vi "Document My VI QuickDrop Plugin.vi"(6 "Variant in":variant, 7 "Shift Pressed?":bool, 8 "error in (no error)":errorcluster, 10 "QD Combo Box Ref":refnum<vi>, 11 "QD Launch VI Ref":refnum<vi>) -> (0 "error out":errorcluster, 4 "Variant out":variant)   [LabVIEW 2014]
doc: "This VI allows the VI Description Tool to be used with the Quick Drop Frame work\n\nDefault Shortcut - [A]"
uses:
  <userlib>/GA/VI Documentation Tool/TYPE_Version Status.ctl
panel:
  in  "Undo Name":string="Quick Drop Keyboard Shortcut"
  # "Do not change the connector pane of this VI.\n\nSee the block diagram for directions on how to use this template."
  # "Specify the name of the Undo transaction"
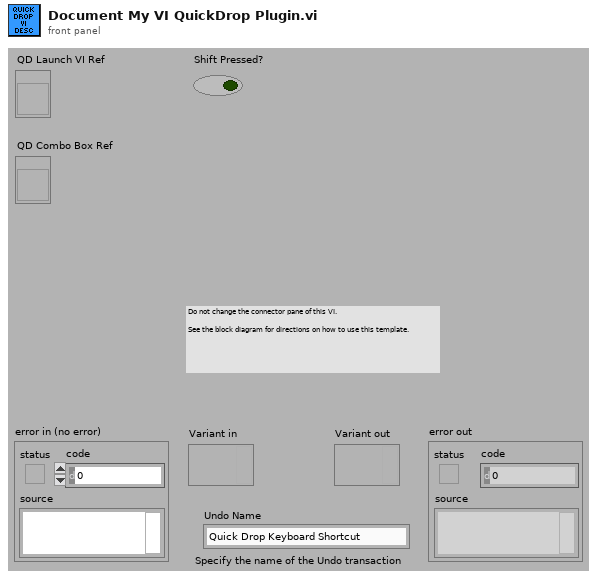
[diagram p1: front panel]
types:
  T1 = typedef "TYPE_Version Status.ctl" = enum16{"Development", "alpha", "beta", "Reviewed", "Bug", "Other"}
  T2 = typedef "TYPE_Description Cluster.ctl" = cluster{"VI Description":string, "VI Version":string, "Review Date":string, "Author":string, "Copyright":string, "Requirements Coverage":string}
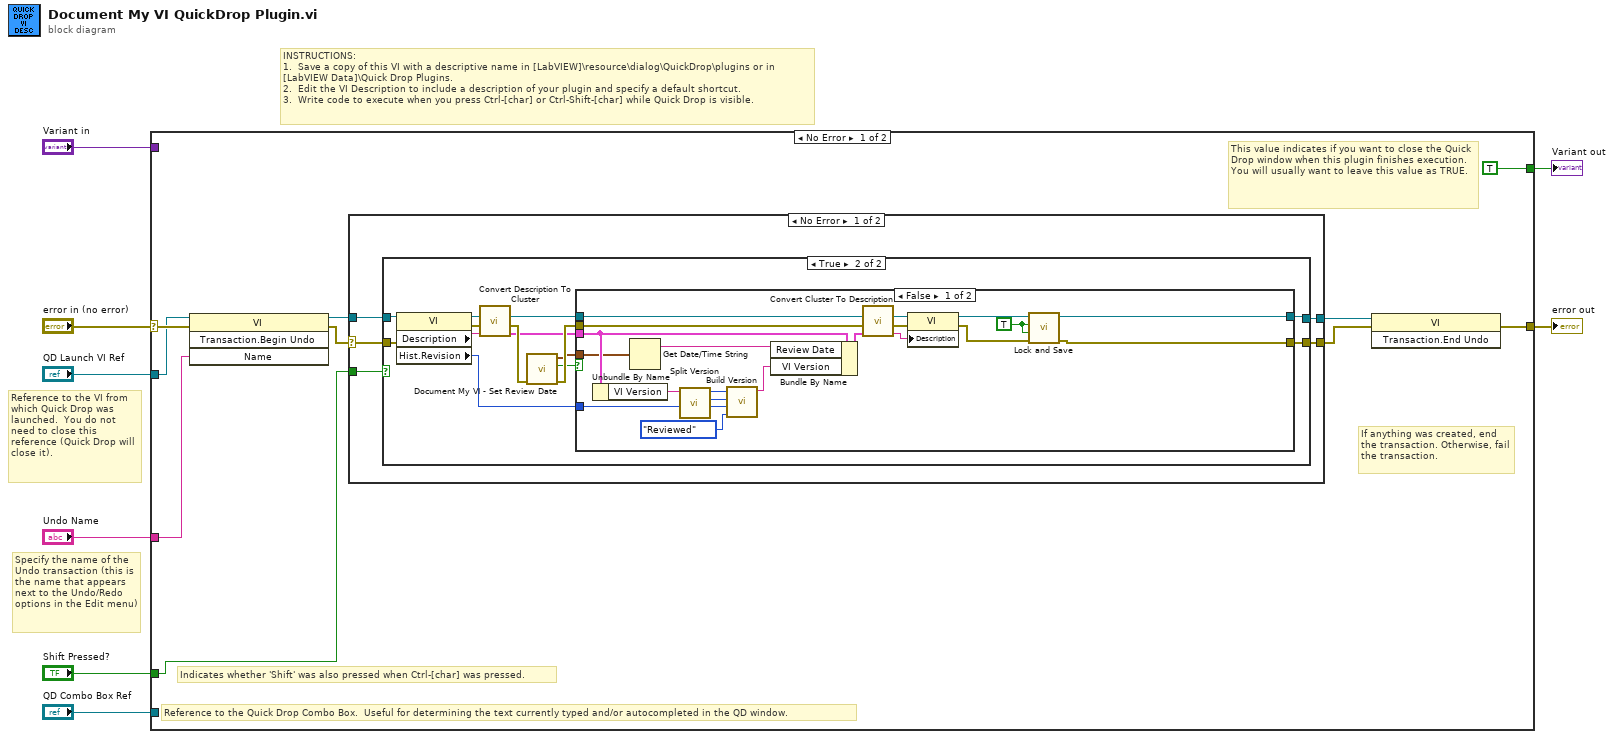
[diagram p0: block diagram]
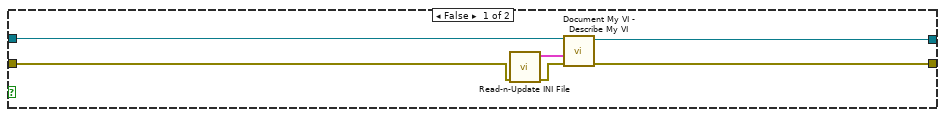
[diagram p2: hidden frame]
diagram:
  # "Specify the name of the Undo transaction (this is the name that appears next to the Undo/Redo options in the Edit menu)"
  # "Reference to the VI from which Quick Drop was launched.  You do not need to close this reference (Quick Drop will close it)."
  # "INSTRUCTIONS:\n1.  Save a copy of this VI with a descriptive name in [LabVIEW]\\resource\\dialog\\QuickDrop\\plugins or in [LabVIEW Data]\\Quick Drop Plugins.\n2.  Edit the VI Description to include a description of your plugin and specify a default shortcut. \n3.  Write code to execute when you press Ctrl-[char] or Ctrl-Shift-[char] while Quick Drop is visible."
  n1 = case shown="No Error" "error in (no error)" {
    selector: "error in (no error)" -> [w18 w66]
    tunnel: [w14 w66] -> w7
    tunnel: "QD Launch VI Ref" -> [w17 _]
    tunnel: "Shift Pressed?" -> [w9 _]
    tunnel: "QD Combo Box Ref" -> [_ _]
    tunnel: "Variant in" -> [_ _]
    tunnel: "Undo Name" -> [w16 _]
    tunnel: [TRUE _] -> w1
    frame No Error {
      # "If anything was created, end the transaction. Otherwise, fail the transaction."
      # "This value indicates if you want to close the Quick Drop window when this plugin finishes execution.  You will usually want to leave this value as TRUE."
      # "Reference to the Quick Drop Combo Box.  Useful for determining the text currently typed and/or autocompleted in the QD window."
      # "Indicates whether 'Shift' was also pressed when Ctrl-[char] was pressed."
      n2 = invoke class="VI" method="Transaction.Begin Undo"(reference=w17, error in=w18, "Name"=w16) -> (reference out=w13:refnum<vi>, error out=w10:errorcluster)  [unwired: 1 in, 2 out]
      n3 = case shown="No Error" w10 {
        selector: w10 -> [w20 w65]
        tunnel: w13 -> [w23 w64]
        tunnel: [w22 w65] -> w12
        tunnel: [w21 w64] -> w11
        tunnel: w9 -> [w19 _]
        frame No Error {
          n4 = case shown="True" w19 {
            tunnel: w23 -> [w29 w41]
            tunnel: [w28 w36] -> w22
            tunnel: [w25 w37] -> w21
            tunnel: w20 -> [w24 w42]
            frame False {
              n5 = call <userlib>:"Read-n-Update INI File.vi"("error in (no error)"=w24) -> ("error out"=w26:errorcluster, "Config Data Out"=w27:cluster{"Company":string, "Author":string})  [unwired: 9 in]
              n6 = call <userlib>:"Document My VI - Describe My VI.vi"("error in (no error)"=w26, "Config Data"=w27, "Active VI Ref In"=w29) -> ("error out"=w28:errorcluster, "Active VI Ref Out"=w25:refnum<vi>)  [unwired: 7 in]
            }
            frame True {
              n7 = property class="VI"(reference=w41, error in=w42) -> (reference out=w38:refnum<vi>, error out=w39:errorcluster, "Description"=w40:string, "Hist.Revision"=w30:u32)
              n8 = call <userlib>:"Convert Description To Cluster.vi"("Description String (empty)"=w40, "error in (no error)"=w39) -> ("Description Cluster"=w32:T2, "error out"=w35:errorcluster)  [unwired: 8 in]
              n9 = call <userlib>:"Document My VI - Set Review Date.vi"("error in (no error)"=w35) -> ("error out"=w34:errorcluster, "Canceled"=w33:bool, "Date of Review out"=w31:timestamp)  [unwired: 8 in]
              n10 = case shown="False" w33 {
                tunnel: w38 -> [w61 w62]
                tunnel: [w46 w62] -> w37
                tunnel: [w44 w63] -> w36
                tunnel: w34 -> [w60 w63]
                tunnel: w32 -> [w56 _]
                tunnel: w31 -> [w51 _]
                tunnel: w30 -> [w48 _]
                frame False {
                  w43 = TRUE ("Lock?")
                  n11 = Unbundle By Name(w56) -> ("VI Version"=w53:string)
                  n12 = Get Date/Time String(seconds (now)=w51) -> (date string=w50:string)  [unwired: 2 in, 1 out]
                  n13 = call <userlib>:"Split Version.vi"("VI Version"=w53) -> ("Minor Version"=w54:u16, "Major Version"=w55:u16)  [unwired: 7 in, 2 out]
                  n14 = call <userlib>:"Build Version.vi"("Current Phase"=TYPE_Version_Status."Reviewed", "Revision"=w48, "Minor Revision"=w54, "Major Revision"=w55) -> ("VI Version"=w52:string)  [unwired: 7 in]
                  n15 = Bundle By Name(cluster=w56, "Review Date"=w50, "VI Version"=w52) -> (w57:T2)
                  n16 = call <userlib>:"Convert Cluster To Description.vi"("Description Cluster"=w57, "error in (no error)"=w60) -> ("Description String (empty)"=w58:string, "error out"=w59:errorcluster)  [unwired: 8 in]
                  n17 = property class="VI"(reference=w61, error in=w59, "Description"=w58) -> (reference out=w47:refnum<vi>, error out=w45:errorcluster)
                  n18 = call <userlib>:"Lock and Save.vi"("error in (no error)"=w45, "Revision Comments?"=w43, "Lock?"=w43, "VI Ref"=w47) -> ("error out"=w44:errorcluster, "VI Ref out"=w46:refnum<vi>)  [unwired: 6 in]
                }
                frame True {
                }
              }
            }
          }
        }
        frame Error {
        }
      }
      n19 = invoke class="VI" method="Transaction.End Undo"(reference=w11, error in=w12) -> (error out=w14:errorcluster)  [unwired: 1 in, 2 out]
    }
    frame Error {
    }
  }
  "error out" <- w7
  "Variant out" <- w1
